vi "Handle Error.vi"(8 "error in (no error)":errorcluster, 11 "KIM101 in":refnum<class "KIM101.lvclass">) -> (0 "error out":errorcluster, 2 "stop actor?":bool=TRUE, 3 "KIM101 out":refnum<class "KIM101.lvclass">)   [LabVIEW 2023, in "KIM101.lvlib" / "KIM101.lvclass"]
doc: "(<B>Filename</B>: Actor Framework.lvlib:Actor.lvclass:Handle Error.vi)\n\nDefines how the actor handles an error that occurred while processing a message. By default, this method does nothing except stop the actor."
uses:
  KIM101.lvclass
  <vilib>/ActorFramework/Actor/Actor.lvclass
  KIM101.lvclass/KIM101.ctl
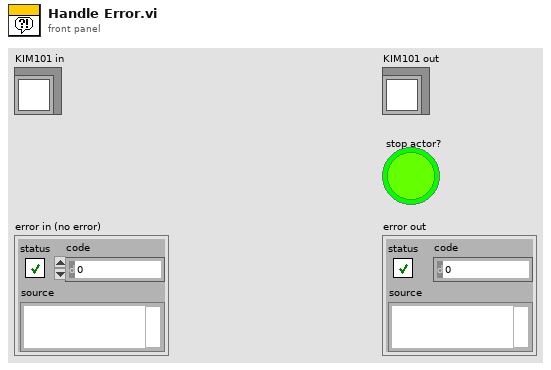
[diagram p1: front panel]
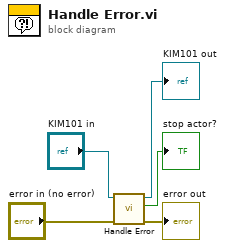
[diagram p0: block diagram]
diagram:
  n1 = call-parent "Handle Error.vi"("error in (no error)"="error in (no error)", "Actor in"="KIM101 in") -> ("error out"=→"error out":errorcluster, "stop actor?"=→"stop actor?":bool, "Actor out"=→"KIM101 out":refnum<class "KIM101.lvclass">)  [unwired: 7 in]
